vi "GetJSONElementValue.vi"(7 "JSON string":string, 10 "JSON element name":string) -> (2 "JSON element value":string, 4 "JSON element found":bool)   [LabVIEW 2013]
uses:
  <vilib>/regexp/Match Regular Expression.xnode
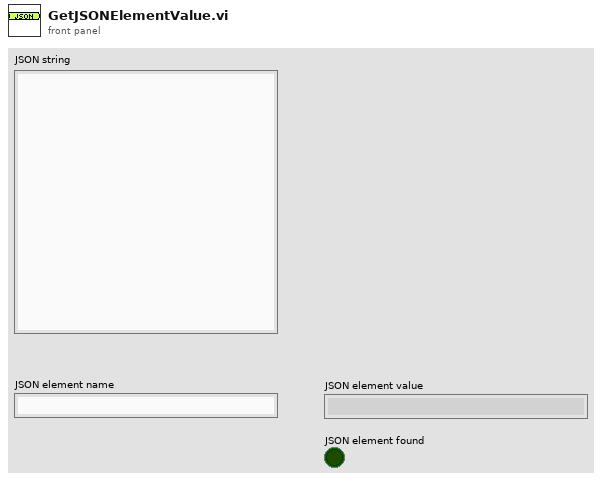
[diagram p1: front panel]
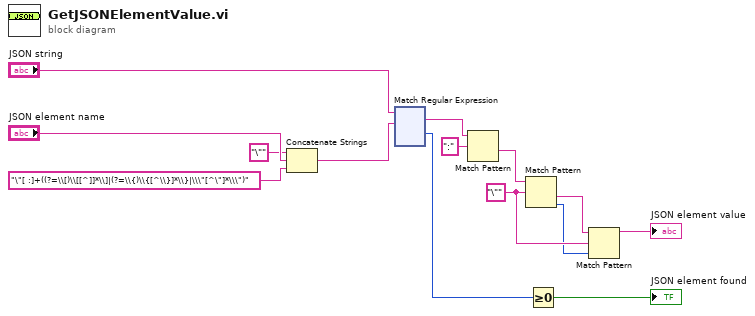
[diagram p0: block diagram]
diagram:
  w8 = "\"" ("regular expression")
  n1 = Concatenate Strings("\"" ("string"), "JSON element name", "\"[ :]+((?=\\[)\\[[^]]*\\]|(?=\\{)\\{[^\\}]*\\}|\\\"[^\"]*\\\")" ("regular expression")) -> (w10:string)
  n2 = xnode "Match Regular Expression"("input string"="JSON string", "regular expression"=w10) -> ("whole match"=w4:string, "offset past match"=w2:i32)  [unwired: 4 in, 3 out]
  n3 = Match Pattern(string=w4, regular expression=":") -> (after substring=w6:string)  [unwired: 1 in, 3 out]
  n4 = Match Pattern(string=w6, regular expression=w8) -> (after substring=w9:string, offset past match=w7:i32)  [unwired: 1 in, 2 out]
  n5 = Greater Or Equal To 0?(x=w2) -> (x >= 0?=→"JSON element found":bool)
  n6 = Match Pattern(string=w9, regular expression=w8, offset (0)=w7) -> (before substring=→"JSON element value":string)  [unwired: 3 out]
